vi "backwash.vi"(4 "Manual override":bool, 6 "Backwash control":T2, 10 "backwash":T1={"Filtered quality target [NTU]"=0.3, "min filtration time [s]"=600.0, "Ripen time [s]"=600.0}, 11 "Filtered Turbidity":dbl) -> (0 "backwashing?":i16, 1 "backwashing?":bool, 3 "last backwash":timestamp)   [LabVIEW 2015]
uses:
  Manual or Auto.ctl
  backwash.ctl
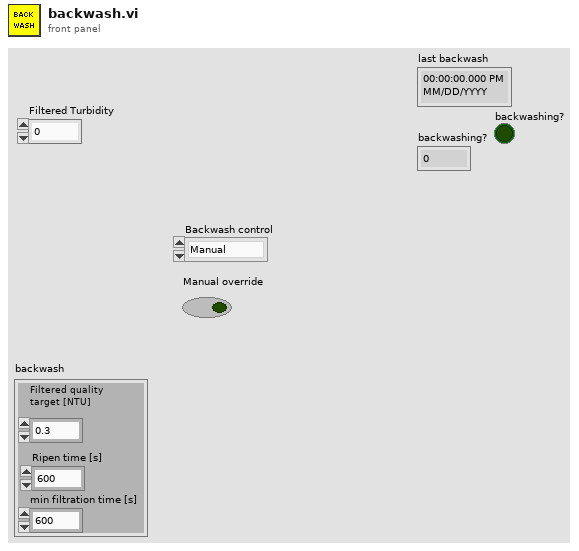
[diagram p1: front panel]
types:
  T1 = typedef "backwash.ctl" = cluster{"Filtered quality target [NTU]":dbl, "min filtration time [s]":dbl, "Ripen time [s]":dbl}
  T2 = typedef "Manual or Auto.ctl" = enum16{"Manual", "Automatic"}
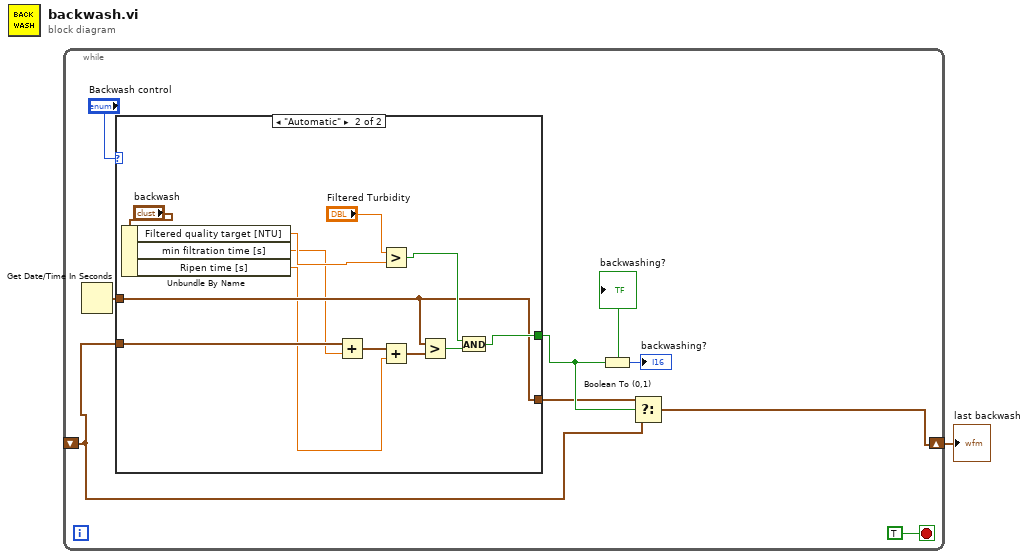
[diagram p0: block diagram]
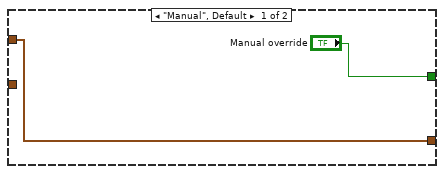
[diagram p2: hidden frame]
diagram:
  n1 = while {
    shift-right: [w8] -> w1
    shift-left: _ -> [w6]
    stop <- TRUE stop-if-true
    n2 = Get Date/Time In Seconds() -> (seconds since 1Jan1904=w5:timestamp)
    n3 = case shown="\"Automatic\"" "Backwash control" {
      tunnel: w6 -> [_ w19]
      tunnel: ["Manual override" w18] -> w3
      tunnel: w5 -> [w10 w16]
      tunnel: [w10 w16] -> w2
      frame "Manual", Default {
      }
      frame "Automatic" {
        n4 = Unbundle By Name("backwash") -> ("Filtered quality target [NTU]"=w14:dbl, "min filtration time [s]"=w13:dbl, "Ripen time [s]"=w12:dbl)
        n5 = Add(x=w19, y=w13) -> (x+y=w22:timestamp)
        n6 = Greater?(x="Filtered Turbidity", y=w14) -> (0:w17:bool)
        n7 = Add(x=w22, y=w12) -> (x+y=w20:timestamp)
        n8 = Greater?(x=w16, y=w20) -> (0:w21:bool)
        n9 = And(x=w17, y=w21) -> (x .and. y?=w18:bool)
      }
    }
    "backwashing?" <- w3
    n10 = Boolean To (0,1)(Boolean=w3) -> (0, 1=→"backwashing?":i16)
    n11 = Select(t=w2, s=w3, f=w6) -> (s? t:f=w8:timestamp)
  }
  "last backwash" <- w1
